vi "TestInstruc.vi"() -> ()   [LabVIEW 2015]
panel:
  in  "Instruction":u8
  in  "Apply":bool
  in  "stop":bool
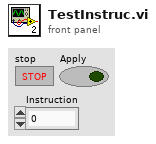
[diagram p1: front panel]
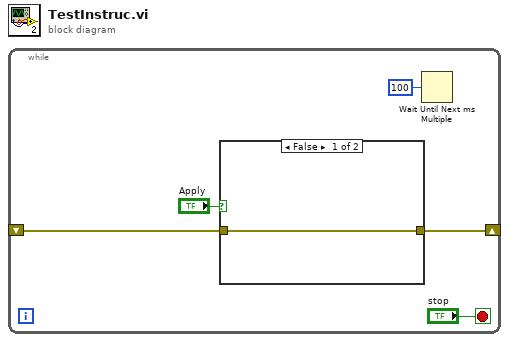
[diagram p0: block diagram]
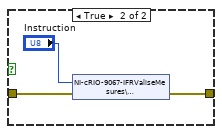
[diagram p2: hidden frame]
diagram:
  n1 = while {
    shift-right: [w3] -> _
    shift-left: _ -> [w2]
    stop <- "stop" stop-if-true
    n2 = case shown="False" "Apply" {
      tunnel: [w6 w9] -> w3
      tunnel: w2 -> [w6 w8]
      frame False {
      }
      frame True {
        n3 = shared-variable "NI-cRIO-9067-IFRValiseMesures\\Bibliothèque2Variables.lvlib\\Instruction"("Instruction", error in=w8) -> (error out=w9:errorcluster)
      }
    }
    n4 = Wait Until Next ms Multiple(millisecond multiple=u32 100) -> ()  [unwired: 1 out]
  }
